vi "test Message - Peek.vi"(8 "error in (no error)":errorcluster, 11 "TestCase in":refnum<class "Test_Queue.lvclass">) -> (0 "error out":errorcluster, 3 "TestCase out":refnum<class "Test_Queue.lvclass">)   [LabVIEW 2015, in "Test_Queue.lvclass"]
uses:
  Test_Queue.lvclass
  Global Parameters.vi
  Core/Session/Session.lvclass
  Queue/NI_Azure_Queue.lvlib
  _shared/_Unit Tests Shared.lvlib
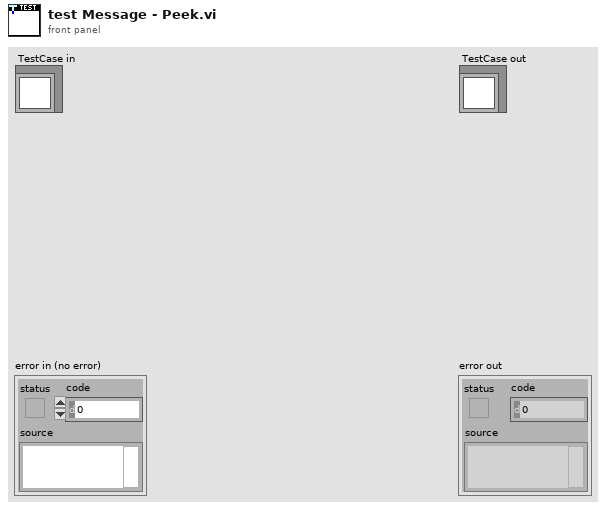
[diagram p1: front panel]
types:
  T1 = typedef "NI_Azure_Core.lvlib/Session.lvclass/Azure Credentials.ctl" = cluster{"Storage Account Name":string, "Access Key":string}
  T2 = typedef "NI_Azure_Queue.lvlib/Message.ctl" = cluster{"Message ID":string, "Insertion Time":string, "Expiration Time":string, "Pop Receipt":string, "Time Next Visible":string, "Dequeue Count":i32, "Message Text":string}
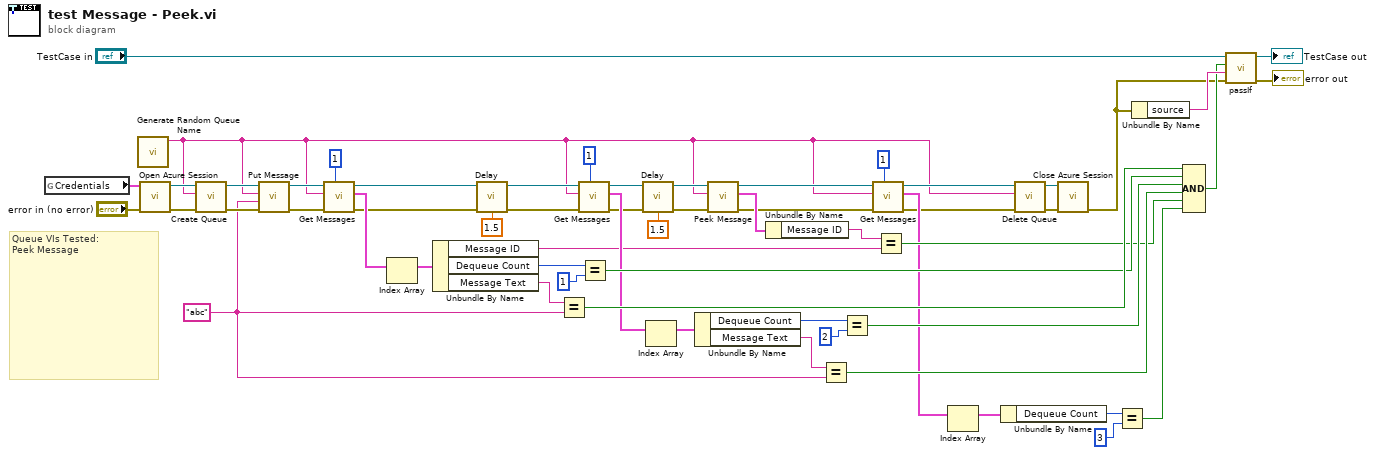
[diagram p0: block diagram]
diagram:
  w26 = "abc" ("Message")
  # "Queue VIs Tested:\nPeek Message"
  n1 = global read "Global Parameters.vi" "Credentials"() -> (w50:T1)
  n2 = call "Generate Random Queue Name.vi"() -> ("Random Queue Name"=w12:string)  [unwired: 11 in]
  n3 = call "Open Azure Session.vi"("error in (no error)"="error in (no error)", "Credentials"=w50) -> ("error out"=w51:errorcluster, "Azure Session"=w46:refnum<class "Session.lvclass">)  [unwired: 8 in]
  n4 = call "Create Queue.vi"("error in (no error)"=w51, "Queue"=w12, "Azure Session in"=w46) -> ("error out"=w47:errorcluster, "Azure Session out"=w42:refnum<class "Session.lvclass">)  [unwired: 7 in]
  n5 = call "Put Message.vi"("error in (no error)"=w47, "Message"=w26, "Queue"=w12, "Azure Session in"=w42) -> ("error out"=w43:errorcluster, "Azure Session out"=w41:refnum<class "Session.lvclass">)  [unwired: 5 in, 1 out]
  n6 = call "Get Messages.vi"("Visibility timeout (30 seconds)"=u32 1, "error in (no error)"=w43, "Queue"=w12, "Azure Session in"=w41) -> ("error out"=w29:errorcluster, "Messages"=w40:T2[], "Azure Session out"=w30:refnum<class "Session.lvclass">)  [unwired: 5 in]
  n7 = Index Array(array=w40) -> (element=w6:T2)  [unwired: 1 in]
  n8 = Unbundle By Name(w6) -> ("Message ID"=w22:string, "Dequeue Count"=w37:i32, "Message Text"=w39:string)
  n9 = call "Delay.vi"("error in"=w29, "delay (1 sec)"=1.5) -> ("error out"=w10:errorcluster)  [unwired: 13 in]
  n10 = Equal?(x=w39, y=w26) -> (x = y?=w38:bool)
  n11 = call "Get Messages.vi"("Visibility timeout (30 seconds)"=u32 1, "error in (no error)"=w10, "Queue"=w12, "Azure Session in"=w30) -> ("error out"=w25:errorcluster, "Messages"=w31:T2[], "Azure Session out"=w24:refnum<class "Session.lvclass">)  [unwired: 5 in]
  n12 = Equal?(x=w37, y=1) -> (x = y?=w35:bool)
  n13 = call "Delay.vi"("error in"=w25, "delay (1 sec)"=1.5) -> ("error out"=w8:errorcluster)  [unwired: 13 in]
  n14 = Index Array(array=w31) -> (element=w5:T2)  [unwired: 1 in]
  n15 = Unbundle By Name(w5) -> ("Dequeue Count"=w33:i32, "Message Text"=w32:string)
  n16 = call "Peek Message.vi"("error in (no error)"=w8, "Queue"=w12, "Azure Session in"=w24) -> ("error out"=w20:errorcluster, "Message"=w23:T2, "Azure Session out"=w19:refnum<class "Session.lvclass">)  [unwired: 6 in]
  n17 = Unbundle By Name(w23) -> ("Message ID"=w11:string)
  n18 = Equal?(x=w32, y=w26) -> (x = y?=w27:bool)
  n19 = Equal?(x=w33, y=2) -> (x = y?=w28:bool)
  n20 = call "Get Messages.vi"("Visibility timeout (30 seconds)"=u32 1, "error in (no error)"=w20, "Queue"=w12, "Azure Session in"=w19) -> ("error out"=w14:errorcluster, "Messages"=w16:T2[], "Azure Session out"=w13:refnum<class "Session.lvclass">)  [unwired: 5 in]
  n21 = Equal?(x=w11, y=w22) -> (x = y?=w21:bool)
  n22 = Index Array(array=w16) -> (element=w4:T2)  [unwired: 1 in]
  n23 = Unbundle By Name(w4) -> ("Dequeue Count"=w17:i32)
  n24 = call "Delete Queue.vi"("error in (no error)"=w14, "Queue"=w12, "Azure Session in"=w13) -> ("error out"=w45:errorcluster, "Azure Session out"=w44:refnum<class "Session.lvclass">)  [unwired: 7 in]
  n25 = call "Close Azure Session.vi"("error in (no error)"=w45, "Azure Session"=w44) -> ("error out"=w48:errorcluster)  [unwired: 9 in]
  n26 = Equal?(x=w17, y=3) -> (x = y?=w15:bool)
  n27 = Unbundle By Name(w48) -> ("source"=w53:string)
  n28 = Compound Arithmetic op=AND(w38, w35, w28, w27, w21, w15) -> (w49:bool)
  n29 = call-dynamic "passIf.vi"("error in (no error)"=w48, "message (\"\")"=w53, "pass"=w49, "TestCase in"="TestCase in") -> ("error out"=→"error out":errorcluster, "TestCase out"=→"TestCase out":refnum<class "Test_Queue.lvclass">)  [unwired: 6 in]
